vi "Create Message Getter.vi"(7 "RPC Message Name":string, 8 "error in (no error)":errorcluster, 11 "RPC Messages Folder (ProjectItem) in":refnum<vi>) -> (0 "error out":errorcluster, 2 "Message Getter out":refnum<vi>, 3 "RPC Messages Folder (ProjectItem) out":refnum<vi>)   [LabVIEW 2019, in "gRPC Scripting Tools.lvlib"]
uses:
  gRPC Scripting Tools.lvlib
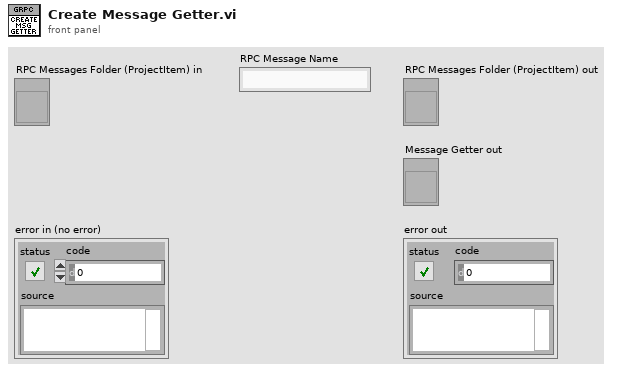
[diagram p1: front panel]
types:
  T1 = enum32{"invalid VI type", "Standard VI", "Control VI", "Global VI", "Polymorphic VI", "Configuration VI", "SubSystem", "Facade VI", "Method VI"}
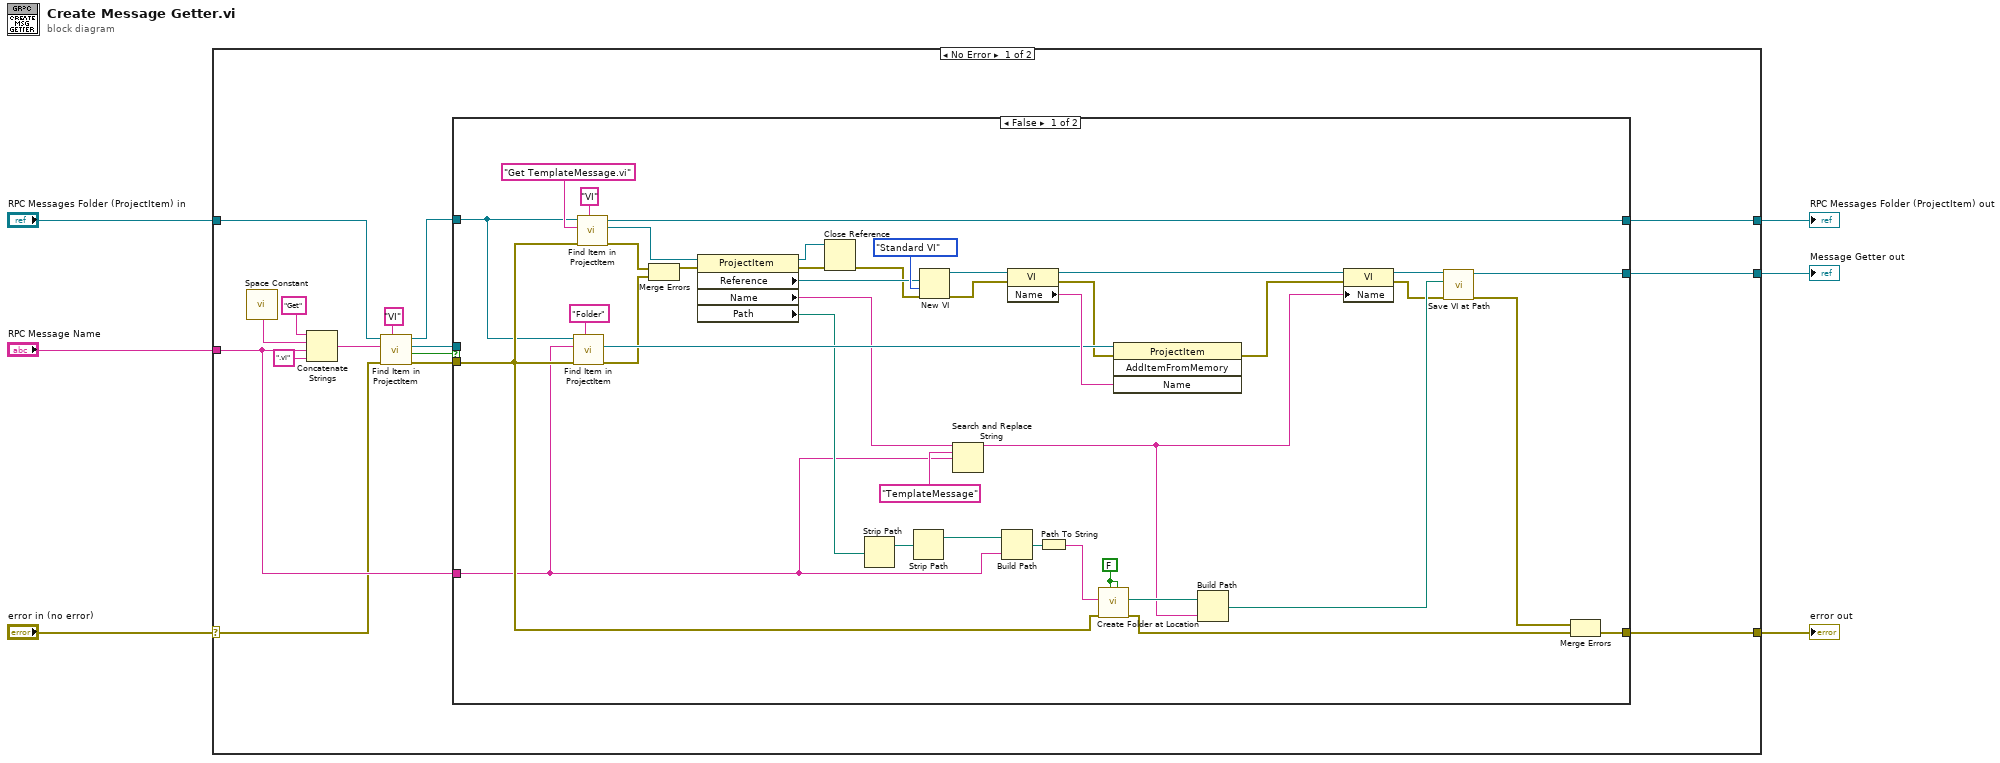
[diagram p0: block diagram]
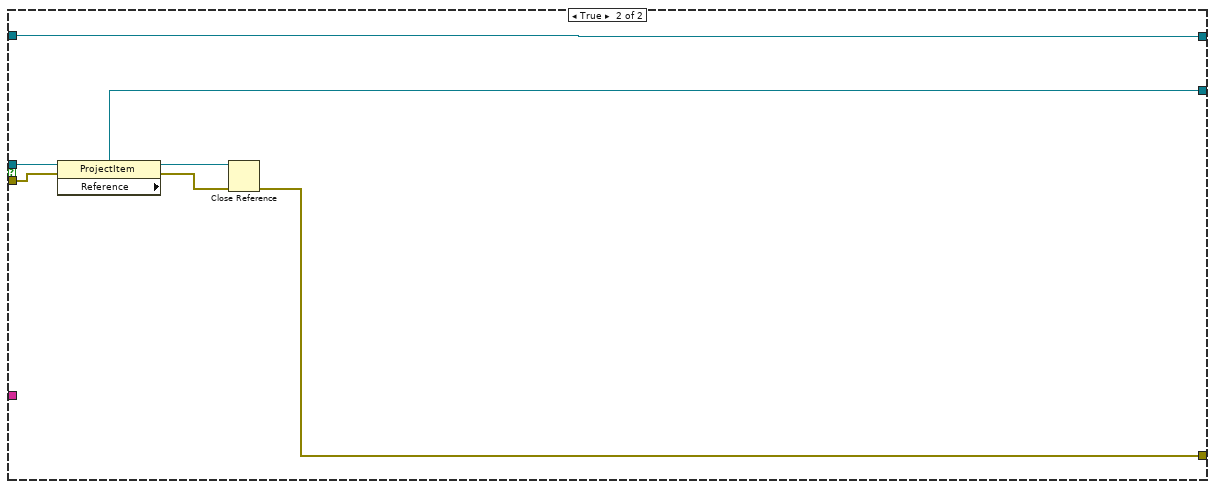
[diagram p2: hidden frame]
diagram:
  n1 = case shown="No Error" "error in (no error)" {
    selector: "error in (no error)" -> [w7 w70]
    tunnel: [w21 _] -> w6
    tunnel: [w20 w69] -> w5
    tunnel: [w19 w70] -> w4
    tunnel: "RPC Messages Folder (ProjectItem) in" -> [w17 w69]
    tunnel: "RPC Message Name" -> [w8 _]
    frame No Error {
      n2 = call <vilib>:"Space Constant.vi"() -> ("String"=w14:string)
      n3 = Concatenate Strings("Get" ("string"), w14, w8, ".vi" ("string")) -> (w12:string)
      n4 = call "Find Item in ProjectItem.vi"("Item Type"="VI", "error in (no error)"=w7, "Name"=w12, "ProjectItem in"=w17) -> ("error out"=w10:errorcluster, "Found ?"=w11:bool, "Item Refnum out"=w9:refnum<vi>, "ProjectItem out"=w16:refnum<vi>)  [unwired: 4 in]
      n5 = case shown="False" w11 {
        tunnel: [w36 w66] -> w21
        tunnel: [w35 w65] -> w20
        tunnel: w10 -> [w30 w67]
        tunnel: [w27 w62] -> w19
        tunnel: w16 -> [w26 w65]
        tunnel: w9 -> [_ w68]
        tunnel: w8 -> [w22 _]
        frame False {
          w34 = FALSE ("Use Relative (F)")
          n6 = call "Find Item in ProjectItem.vi"("Item Type"="Folder", "error in (no error)"=w30, "Name"=w22, "ProjectItem in"=w26) -> ("error out"=w31:errorcluster, "Item Refnum out"=w52:refnum<vi>)  [unwired: 4 in, 2 out]
          n7 = call "Find Item in ProjectItem.vi"("Item Type"="VI", "error in (no error)"=w30, "Name"="Get TemplateMessage.vi", "ProjectItem in"=w26) -> ("error out"=w33:errorcluster, "Item Refnum out"=w58:refnum<vi>, "ProjectItem out"=w35:refnum<vi>)  [unwired: 4 in, 1 out]
          n8 = Merge Errors(w33, w31) -> (w32:errorcluster)
          n9 = property class="ProjectItem"(reference=w58, error in=w32) -> (reference out=w23:refnum<vi>, error out=w25:errorcluster, "Reference"=w54:refnum<vi>, "Name"=w45:string, "Path"=w47:path)
          n10 = Close Reference(reference=w23, error in (no error)=w25) -> (error out=w24:errorcluster)
          n11 = Strip Path(path=w47) -> (stripped path=w51:path)  [unwired: 1 out]
          n12 = Strip Path(path=w51) -> (stripped path=w50:path)  [unwired: 1 out]
          n13 = New VI(8:w24, 9:T1."Standard VI" ("vi type (standard vi)"), 10:w54) -> (0:w55:errorcluster, 3:w57:refnum<vi>)  [unwired: 1 in, 3 out]
          n14 = Search and Replace String(input string=w45, search string="TemplateMessage", replace string=w22) -> (result string=w40:string)  [unwired: 5 in, 3 out]
          n15 = Build Path(base path=w50, name or relative path=w22) -> (appended path=w49:path)
          n16 = property class="VI"(reference=w57, error in=w55) -> (reference out=w44:refnum<vi>, error out=w43:errorcluster, "Name"=w53:string)
          n17 = Path To String(path=w49) -> (string=w48:string)
          n18 = call "Create Folder at Location.vi"("Override existing (F)"=w34, "Use Relative (F)"=w34, "Error In"=w30, "Path"=w48) -> ("Error Out"=w29:errorcluster, "Full path out"=w41:path)  [unwired: 5 in, 1 out]
          n19 = invoke class="ProjectItem" method="AddItemFromMemory"(reference=w52, error in=w43, "Name"=w53) -> (error out=w42:errorcluster)  [unwired: 1 in, 3 out]
          n20 = Build Path(base path=w41, name or relative path=w40) -> (appended path=w38:path)
          n21 = property class="VI"(reference=w44, error in=w42, "Name"=w40) -> (reference out=w39:refnum<vi>, error out=w37:errorcluster)
          n22 = call "Save VI at Path.vi"("error in (no error)"=w37, "Path"=w38, "VI in"=w39) -> ("error out"=w28:errorcluster, "VI out"=w36:refnum<vi>)  [unwired: 6 in, 1 out]
          n23 = Merge Errors(w28, w29) -> (w27:errorcluster)
        }
        frame True {
          n24 = property class="ProjectItem"(reference=w68, error in=w67) -> (reference out=w63:refnum<vi>, error out=w64:errorcluster, "Reference"=w66:refnum<vi>)
          n25 = Close Reference(reference=w63, error in (no error)=w64) -> (error out=w62:errorcluster)
        }
      }
    }
    frame Error {
    }
  }
  "error out" <- w4
  "Message Getter out" <- w6
  "RPC Messages Folder (ProjectItem) out" <- w5
